vi "velPlanningMultipleDests.vi"(5 "delta":dbl, 6 "v_desired":dbl, 7 "V_sent":dbl=3.0 format="%#_13g", 8 "error in (no error)":errorcluster, 9 "Dests":dbl[][](array[numeric]), 10 "Robot":refnum<class "Robot.lvclass">, 11 "Game in":refnum<class "Game.lvclass">) -> (0 "error out":errorcluster, 1 "v_desired_for_dest":dbl, 2 "dest":dbl[](array[numeric]), 3 "Game out":refnum<class "Game.lvclass">)   [LabVIEW 2020, in "Game.lvclass"]
uses:
  Game.lvclass
  Robot_class/Robot.lvclass
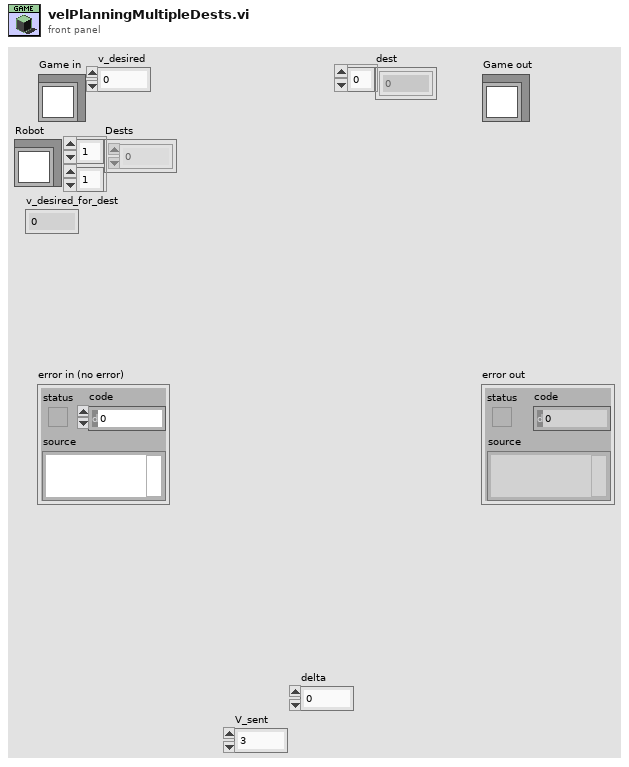
[diagram p1: front panel]
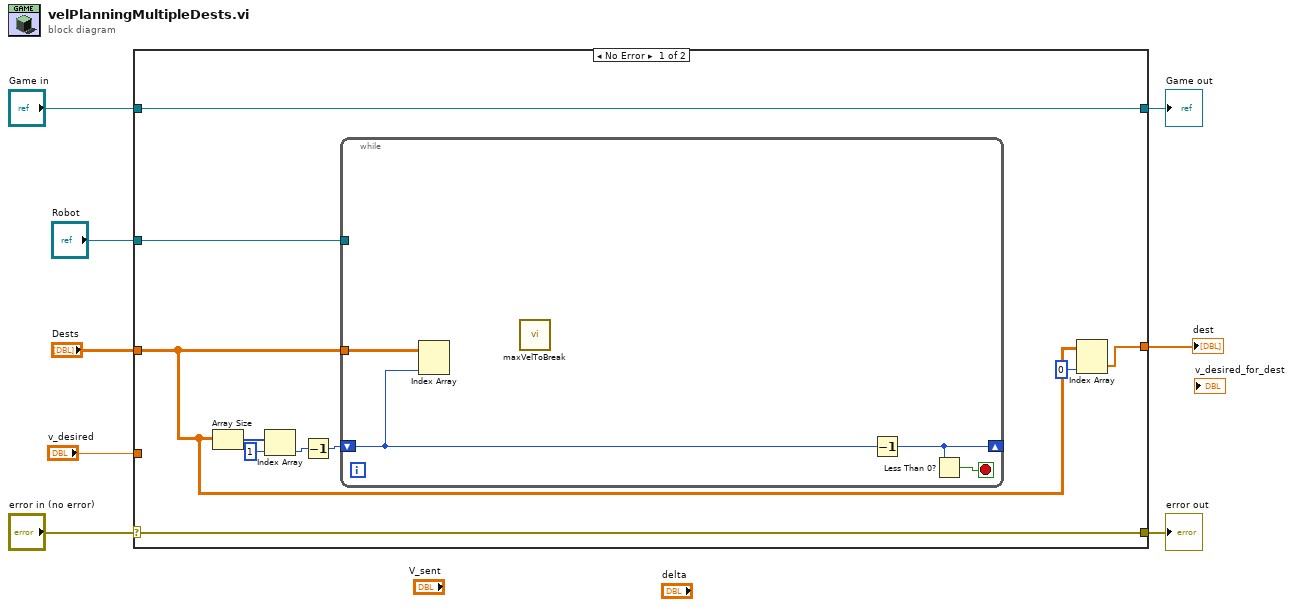
[diagram p0: block diagram]
diagram:
  n1 = case shown="No Error" "error in (no error)" {
    selector: "error in (no error)" -> [w17 w24]
    tunnel: [w17 w24] -> w7
    tunnel: [w18 w23] -> w5
    tunnel: "Game in" -> [w18 w23]
    tunnel: "Robot" -> [w12 _]
    tunnel: "Dests" -> [w11 _]
    tunnel: "v_desired" -> [_ _]
    tunnel: [w9 _] -> w1
    frame No Error {
      n2 = Array Size(array=w11) -> (size(s)=w16:i32[])
      n3 = Index Array(array=w16, index=1) -> (element=w14:i32)
      n4 = Decrement(x=w14) -> (x-1=w13:i32)
      n5 = while {
        shift-right: [w21] -> _
        shift-left: w13 -> [w19]
        tunnel: w11 -> [w20]
        tunnel: w12 -> [_]
        stop <- w22 stop-if-true
        n6 = Index Array(array=w20, index (col)=w19) -> ()  [unwired: 1 in, 1 out]
        n7 = call "maxVelToBreak.vi"() -> ()  [unwired: 17 in, 3 out]
        n8 = Decrement(x=w19) -> (x-1=w21:i32)
        n9 = Less Than 0?(x=w21) -> (x < 0?=w22:bool)
      }
      n10 = Index Array(array=w11, index (col)=0 ("disabled index (col)")) -> (element=w9:dbl[])  [unwired: 1 in]
    }
    frame Error {
    }
  }
  "error out" <- w7
  "Game out" <- w5
  "dest" <- w1
